vi "CRYUpdate Unicode MultCol Listbox.vi"(5 "Interpret as Unicode (T)":bool=TRUE, 8 "Data[]":string[][](array[string])) -> (3 "Data[] Out":string[][](array[string]))   [LabVIEW 2013]
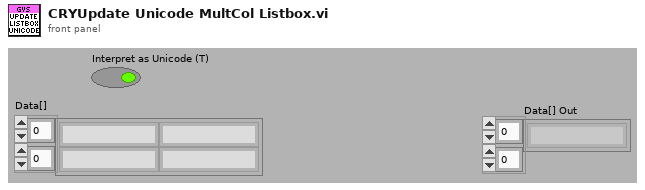
[diagram p1: front panel]
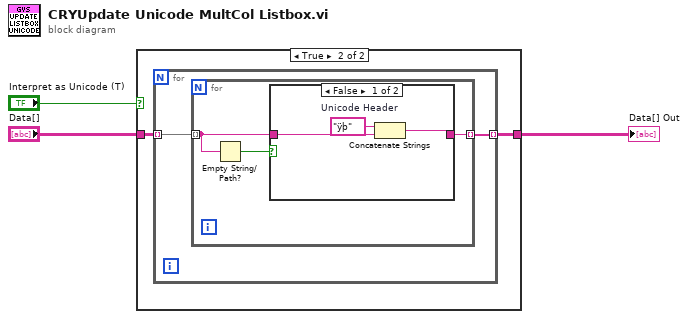
[diagram p0: block diagram]
diagram:
  n1 = case shown="True" "Interpret as Unicode (T)" {
    tunnel: "Data[]" -> [w4 w6]
    tunnel: [w4 w5] -> w1
    frame False {
    }
    frame True {
      n2 = for {
        tunnel: w6 -> [w8] mode=indexing
        tunnel: [w7] -> w5 mode=indexing
        n3 = for {
          tunnel: w8 -> [w10] mode=indexing
          tunnel: [w11] -> w7 mode=indexing
          n4 = Empty String/Path?(string/path=w10) -> (empty?=w9:bool)
          n5 = case shown="False" w9 {
            tunnel: [w12 w15] -> w11
            tunnel: w10 -> [w13 w15]
            frame False {
              w14 = "ÿþ"  # Unicode Header
              n6 = Concatenate Strings(w14, w13) -> (w12:string)
            }
            frame True {
            }
          }
        }
      }
    }
  }
  "Data[] Out" <- w1
